vi "4461 - Create IO Channels Parallel.vi"(6 "AI Buffer Size (s)":i32=10, 8 "sampling info":cluster{"Fs":dbl, "#s":dbl}, 9 "AO":T1={"AO amp (V)"=[0.1, 0.09, 0.08, 0.07, 0.06, 0.05, 0.04, 0.03], "AO DC (V)"=[0.0, 0.0, 0.0, 0.0, 0.0, 0.0, 0.0, 0.0], "AO f (Hz)"=[13.0, 13.0, 13.0, 13.0, 13.0, 13.0, 13.0, 13.0], "AO phi (deg)"=[0.0, 0.0, 0.0, 0.0, 0.0, 0.0, 0.0, 0.0], "function"=[enum."Sine Wave", enum."Sine Wave", enum."Sine Wave", enum."Sine Wave", enum."Sine Wave", enum."Sine Wave", enum."Sine Wave", enum."Sine Wave"]} {"AO DC (V)" format="%#_6p"; "AO amp (V)" format="%#_6p"}, 10 "AO Configuration":T2(array[cluster])=[{"Output physical channels"="PXI1Slot2/ao0", "AO. Max"=0.1, "AO.Min"=-0.1}, {"Output physical channels"="", "AO. Max"=0.1, "AO.Min"=-0.1}], 11 "AI Configuration":T3(array[cluster])=[{"AI.Coupling"=10050, "AI.Max"=10.0, "AI.Min"=-10.0, "Input physical channels"="PXI1Slot2/ai0:1"}, {"AI.Coupling"=10050, "AI.Max"=10.0, "AI.Min"=-10.0, "Input physical channels"="PXI1Slot3/ai0:3"}, {"AI.Coupling"=10050, "AI.Max"=10.0, "AI.Min"=-10.0, "Input physical channels"=""}] {"AI.Coupling" items=["AC"=10045, "DC"=10050, "GND"=10066]}) -> (2 "AO Task":refnum<k21>[](array[refnum]), 3 "AI task":refnum<k21>[](array[refnum]), 4 "phase log":dbl[](array[numeric])=[0.99999999999938, 0.99999999999938], 5 "appended array":errorcluster[][](array[cluster]))   [LabVIEW 2013]
uses:
  <vilib>/DAQmx/configure/timing.llb/DAQmx Timing (Sample Clock).vi
  <vilib>/DAQmx/create/channels.llb/DAQmx Create Channel (AI-Voltage-Basic).vi
  <vilib>/DAQmx/write.llb/DAQmx Write (Analog 1D Wfm NChan NSamp).vi
  <resource>/objmgr/daqmx.rc
  <vilib>/DAQmx/configure/trigger.llb/DAQmx Start Trigger (Digital Edge).vi
  <vilib>/DAQmx/create/channels.llb/DAQmx Create Channel (AO-Voltage-Basic).vi
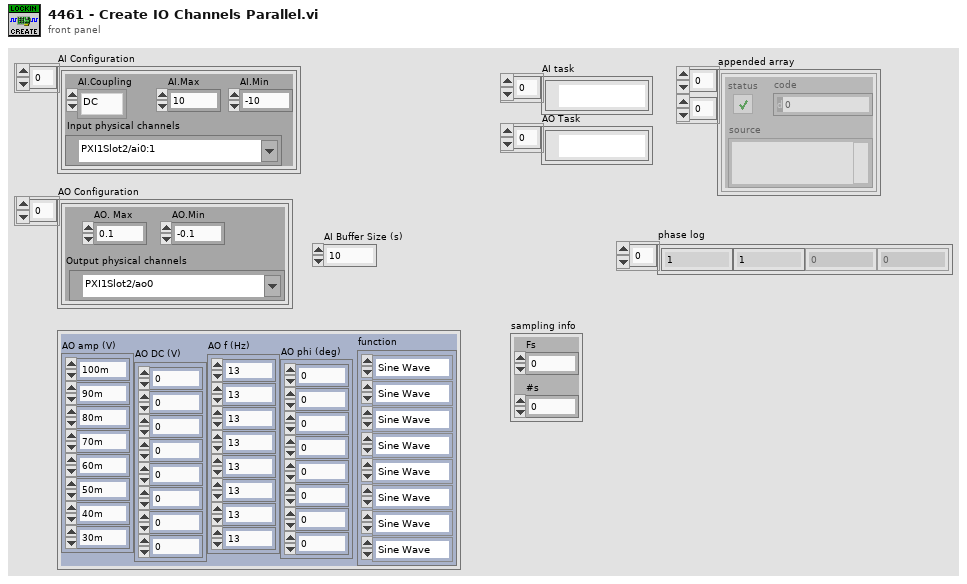
[diagram p1: front panel]
types:
  T1 = cluster{"AO amp (V)":dbl[], "AO DC (V)":dbl[], "AO f (Hz)":dbl[], "AO phi (deg)":dbl[], "function":enum16{"Sine Wave", "Triangle Wave", "Square Wave", "Sawtooth Wave"}[]}
  T2 = cluster{"Output physical channels":tag, "AO. Max":dbl, "AO.Min":dbl}[]
  T3 = cluster{"AI.Coupling":i32, "AI.Max":dbl, "AI.Min":dbl, "Input physical channels":tag}[]
  T4 = cluster{"AI.Coupling":i32, "AI.Max":dbl, "AI.Min":dbl, "Input physical channels":tag}
  T5 = cluster{"Output physical channels":tag, "AO. Max":dbl, "AO.Min":dbl}
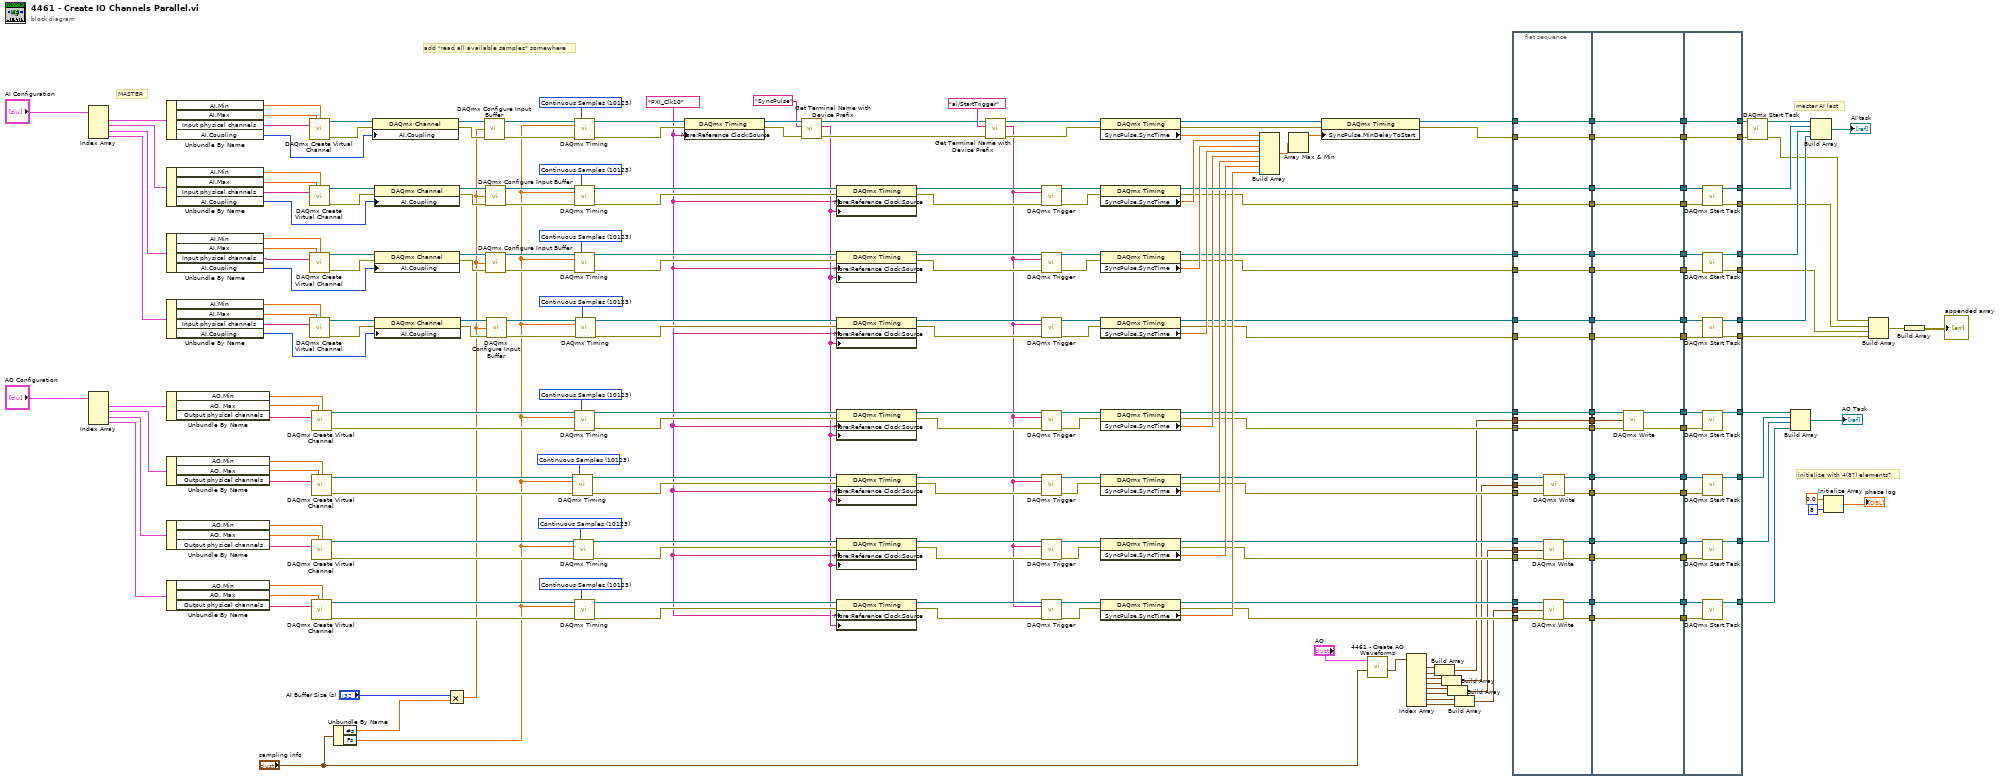
[diagram p0: block diagram]
diagram:
  w23 = tag "PXI_Clk10" ("RefClk.Src")
  w96 = 10123 items=["Finite Samples"=10178, "Continuous Samples"=10123] ("sample mode")
  w111 = 10123 items=["Finite Samples"=10178, "Continuous Samples"=10123] ("sample mode")
  w120 = 10123 items=["Finite Samples"=10178, "Continuous Samples"=10123] ("sample mode")
  w134 = 10123 items=["Finite Samples"=10178, "Continuous Samples"=10123] ("sample mode")
  w161 = 10123 items=["Finite Samples"=10178, "Continuous Samples"=10123] ("sample mode")
  w177 = 10123 items=["Finite Samples"=10178, "Continuous Samples"=10123] ("sample mode")
  w190 = 10123 items=["Finite Samples"=10178, "Continuous Samples"=10123] ("sample mode")
  w229 = 10123 items=["Finite Samples"=10178, "Continuous Samples"=10123] ("sample mode")
  # "master AI last"
  # "initialize with 4(8?) elements?"
  # "add \"read all available samples\" somewhere"
  # "MASTER"
  n1 = Index Array(array="AI Configuration") -> (element #1=w230:T4, element #2=w191:T4, element #3=w154:T4, element #4=w153:T4)  [unwired: 4 in]
  n2 = Index Array(array="AO Configuration") -> (element #1=w138:T5, element #2=w89:T5, element #3=w90:T5, element #4=w91:T5)  [unwired: 4 in]
  n3 = Unbundle By Name(w230) -> ("AI.Min"=w202:dbl, "AI.Max"=w203:dbl, "Input physical channels"=w214:tag, "AI.Coupling"=w201:i32)
  n4 = Unbundle By Name(w191) -> ("AI.Min"=w198:dbl, "AI.Max"=w197:dbl, "Input physical channels"=w192:tag, "AI.Coupling"=w199:i32)
  n5 = Unbundle By Name(w154) -> ("AI.Min"=w170:dbl, "AI.Max"=w171:dbl, "Input physical channels"=w176:tag, "AI.Coupling"=w169:i32)
  n6 = Unbundle By Name(w153) -> ("AI.Min"=w167:dbl, "AI.Max"=w166:dbl, "Input physical channels"=w162:tag, "AI.Coupling"=w168:i32)
  n7 = Unbundle By Name(w138) -> ("AO.Min"=w135:dbl, "AO. Max"=w136:dbl, "Output physical channels"=w137:tag)
  n8 = Unbundle By Name(w89) -> ("AO.Min"=w118:dbl, "AO. Max"=w117:dbl, "Output physical channels"=w116:tag)
  n9 = Unbundle By Name(w90) -> ("AO.Min"=w113:dbl, "AO. Max"=w114:dbl, "Output physical channels"=w115:tag)
  n10 = Unbundle By Name(w91) -> ("AO.Min"=w94:dbl, "AO. Max"=w93:dbl, "Output physical channels"=w92:tag)
  n11 = call-poly <vilib>:"DAQmx Create Virtual Channel.vi"("maximum value"=w203, "minimum value"=w202, "physical channels"=w214) -> ("task out"=w213:refnum<k21>, "error out"=w212:errorcluster)  [unwired: 11 in]
  n12 = call-poly <vilib>:"DAQmx Create Virtual Channel.vi"("maximum value"=w197, "minimum value"=w198, "physical channels"=w192) -> ("task out"=w193:refnum<k21>, "error out"=w194:errorcluster)  [unwired: 11 in]
  n13 = call-poly <vilib>:"DAQmx Create Virtual Channel.vi"("maximum value"=w171, "minimum value"=w170, "physical channels"=w176) -> ("task out"=w175:refnum<k21>, "error out"=w174:errorcluster)  [unwired: 11 in]
  n14 = call-poly <vilib>:"DAQmx Create Virtual Channel.vi"("maximum value"=w166, "minimum value"=w167, "physical channels"=w162) -> ("task out"=w163:refnum<k21>, "error out"=w164:errorcluster)  [unwired: 11 in]
  n15 = call-poly <vilib>:"DAQmx Create Virtual Channel.vi"("maximum value"=w136, "minimum value"=w135, "physical channels"=w137) -> ("task out"=w21:refnum<k21>, "error out"=w20:errorcluster)  [unwired: 11 in]
  n16 = call-poly <vilib>:"DAQmx Create Virtual Channel.vi"("maximum value"=w117, "minimum value"=w118, "physical channels"=w116) -> ("task out"=w119:refnum<k21>, "error out"=w121:errorcluster)  [unwired: 11 in]
  n17 = call-poly <vilib>:"DAQmx Create Virtual Channel.vi"("maximum value"=w114, "minimum value"=w113, "physical channels"=w115) -> ("task out"=w112:refnum<k21>, "error out"=w110:errorcluster)  [unwired: 11 in]
  n18 = call-poly <vilib>:"DAQmx Create Virtual Channel.vi"("maximum value"=w93, "minimum value"=w94, "physical channels"=w92) -> ("task out"=w95:refnum<k21>, "error out"=w97:errorcluster)  [unwired: 11 in]
  n19 = Unbundle By Name("sampling info") -> ("#s"=w2:dbl, "Fs"=w1:dbl)
  n20 = property class="DAQmx Channel"(reference=w213, error in=w212, "AI.Coupling"=w201) -> (reference out=w211:refnum<k21>, error out=w210:errorcluster)
  n21 = property class="DAQmx Channel"(reference=w193, error in=w194, "AI.Coupling"=w199) -> (reference out=w195:refnum<k21>, error out=w196:errorcluster)
  n22 = property class="DAQmx Channel"(reference=w175, error in=w174, "AI.Coupling"=w169) -> (reference out=w173:refnum<k21>, error out=w172:errorcluster)
  n23 = property class="DAQmx Channel"(reference=w163, error in=w164, "AI.Coupling"=w168) -> (reference out=w165:refnum<k21>, error out=w28:errorcluster)
  n24 = Multiply(x="AI Buffer Size (s)", y=w2) -> (x*y=w7:dbl)
  n25 = call <vilib>:"DAQmx Configure Input Buffer.vi"("task/channels in"=w211, "buffer size (in samples per channel)"=w7, "error in"=w210) -> ("task out"=w209:refnum<k21>, "error out"=w208:errorcluster)  [unwired: 11 in]
  n26 = call <vilib>:"DAQmx Configure Input Buffer.vi"("task/channels in"=w195, "buffer size (in samples per channel)"=w7, "error in"=w196) -> ("task out"=w189:refnum<k21>, "error out"=w188:errorcluster)  [unwired: 11 in]
  n27 = call <vilib>:"DAQmx Configure Input Buffer.vi"("task/channels in"=w173, "buffer size (in samples per channel)"=w7, "error in"=w172) -> ("task out"=w178:refnum<k21>, "error out"=w179:errorcluster)  [unwired: 11 in]
  n28 = call <vilib>:"DAQmx Configure Input Buffer.vi"("task/channels in"=w165, "buffer size (in samples per channel)"=w7, "error in"=w28) -> ("task out"=w160:refnum<k21>, "error out"=w159:errorcluster)  [unwired: 11 in]
  n29 = call-poly <vilib>:"DAQmx Timing.vi"("task/channels in"=w119, "sample mode"=w120, "rate"=w1, "error in"=w121) -> ("task out"=w123:refnum<k21>, "error out"=w124:errorcluster)  [unwired: 10 in]
  n30 = call-poly <vilib>:"DAQmx Timing.vi"("task/channels in"=w112, "sample mode"=w111, "rate"=w1, "error in"=w110) -> ("task out"=w108:refnum<k21>, "error out"=w107:errorcluster)  [unwired: 10 in]
  n31 = call-poly <vilib>:"DAQmx Timing.vi"("task/channels in"=w209, "sample mode"=w229, "rate"=w1, "error in"=w208) -> ("task out"=w228:refnum<k21>, "error out"=w200:errorcluster)  [unwired: 10 in]
  n32 = call-poly <vilib>:"DAQmx Timing.vi"("task/channels in"=w189, "sample mode"=w190, "rate"=w1, "error in"=w188) -> ("task out"=w187:refnum<k21>, "error out"=w186:errorcluster)  [unwired: 10 in]
  n33 = call-poly <vilib>:"DAQmx Timing.vi"("task/channels in"=w178, "sample mode"=w177, "rate"=w1, "error in"=w179) -> ("task out"=w180:refnum<k21>, "error out"=w181:errorcluster)  [unwired: 10 in]
  n34 = call-poly <vilib>:"DAQmx Timing.vi"("task/channels in"=w21, "sample mode"=w134, "rate"=w1, "error in"=w20) -> ("task out"=w132:refnum<k21>, "error out"=w131:errorcluster)  [unwired: 10 in]
  n35 = call-poly <vilib>:"DAQmx Timing.vi"("task/channels in"=w95, "sample mode"=w96, "rate"=w1, "error in"=w97) -> ("task out"=w99:refnum<k21>, "error out"=w100:errorcluster)  [unwired: 10 in]
  n36 = call-poly <vilib>:"DAQmx Timing.vi"("task/channels in"=w160, "sample mode"=w161, "rate"=w1, "error in"=w159) -> ("task out"=w158:refnum<k21>, "error out"=w157:errorcluster)  [unwired: 10 in]
  n37 = property class="DAQmx Timing"(reference=w228, error in=w200, "More:Reference Clock:Source"=w23) -> (reference out=w27:refnum<k21>, error out=w26:errorcluster)
  n38 = call "Get Terminal Name with Device Prefix.vi"("error in (no error)"=w26, "Local Terminal Name"="SyncPulse", "task/channels in"=w27) -> ("error out"=w223:errorcluster, "Terminal Name with Device Prefix"=w24:tag, "task out"=w224:refnum<k21>)  [unwired: 6 in]
  n39 = property class="DAQmx Timing"(reference=w187, error in=w186, "More:Reference Clock:Source"=w23, "More:Synchronization Pulse:Source"=w24) -> (reference out=w185:refnum<k21>, error out=w184:errorcluster)
  n40 = property class="DAQmx Timing"(reference=w180, error in=w181, "More:Reference Clock:Source"=w23, "More:Synchronization Pulse:Source"=w24) -> (reference out=w182:refnum<k21>, error out=w183:errorcluster)
  n41 = property class="DAQmx Timing"(reference=w158, error in=w157, "More:Reference Clock:Source"=w23, "More:Synchronization Pulse:Source"=w24) -> (reference out=w156:refnum<k21>, error out=w155:errorcluster)
  n42 = property class="DAQmx Timing"(reference=w132, error in=w131, "More:Reference Clock:Source"=w23, "More:Synchronization Pulse:Source"=w24) -> (reference out=w133:refnum<k21>, error out=w130:errorcluster)
  n43 = property class="DAQmx Timing"(reference=w123, error in=w124, "More:Reference Clock:Source"=w23, "More:Synchronization Pulse:Source"=w24) -> (reference out=w122:refnum<k21>, error out=w125:errorcluster)
  n44 = property class="DAQmx Timing"(reference=w108, error in=w107, "More:Reference Clock:Source"=w23, "More:Synchronization Pulse:Source"=w24) -> (reference out=w109:refnum<k21>, error out=w106:errorcluster)
  n45 = property class="DAQmx Timing"(reference=w99, error in=w100, "More:Reference Clock:Source"=w23, "More:Synchronization Pulse:Source"=w24) -> (reference out=w98:refnum<k21>, error out=w101:errorcluster)
  n46 = call "Get Terminal Name with Device Prefix.vi"("error in (no error)"=w223, "Local Terminal Name"="ai/StartTrigger", "task/channels in"=w224) -> ("error out"=w221:errorcluster, "Terminal Name with Device Prefix"=w84:tag, "task out"=w222:refnum<k21>)  [unwired: 6 in]
  n47 = call-poly <vilib>:"DAQmx Trigger.vi"("task/channels in"=w185, "source"=w84, "error in"=w184) -> ("task out"=w150:refnum<k21>, "error out"=w149:errorcluster)  [unwired: 11 in]
  n48 = call-poly <vilib>:"DAQmx Trigger.vi"("task/channels in"=w182, "source"=w84, "error in"=w183) -> ("task out"=w151:refnum<k21>, "error out"=w148:errorcluster)  [unwired: 11 in]
  n49 = call-poly <vilib>:"DAQmx Trigger.vi"("task/channels in"=w156, "source"=w84, "error in"=w155) -> ("task out"=w152:refnum<k21>, "error out"=w147:errorcluster)  [unwired: 11 in]
  n50 = call-poly <vilib>:"DAQmx Trigger.vi"("task/channels in"=w133, "source"=w84, "error in"=w130) -> ("task out"=w129:refnum<k21>, "error out"=w128:errorcluster)  [unwired: 11 in]
  n51 = call-poly <vilib>:"DAQmx Trigger.vi"("task/channels in"=w122, "source"=w84, "error in"=w125) -> ("task out"=w126:refnum<k21>, "error out"=w127:errorcluster)  [unwired: 11 in]
  n52 = call-poly <vilib>:"DAQmx Trigger.vi"("task/channels in"=w109, "source"=w84, "error in"=w106) -> ("task out"=w105:refnum<k21>, "error out"=w104:errorcluster)  [unwired: 11 in]
  n53 = call-poly <vilib>:"DAQmx Trigger.vi"("task/channels in"=w98, "source"=w84, "error in"=w101) -> ("task out"=w102:refnum<k21>, "error out"=w103:errorcluster)  [unwired: 11 in]
  n54 = property class="DAQmx Timing"(reference=w222, error in=w221) -> (reference out=w218:refnum<k21>, error out=w219:errorcluster, "SyncPulse.SyncTime"=w220:dbl)
  n55 = property class="DAQmx Timing"(reference=w150, error in=w149) -> (reference out=w140:refnum<k21>, error out=w75:errorcluster, "SyncPulse.SyncTime"=w145:dbl)
  n56 = property class="DAQmx Timing"(reference=w151, error in=w148) -> (reference out=w81:refnum<k21>, error out=w72:errorcluster, "SyncPulse.SyncTime"=w144:dbl)
  n57 = property class="DAQmx Timing"(reference=w152, error in=w147) -> (reference out=w78:refnum<k21>, error out=w69:errorcluster, "SyncPulse.SyncTime"=w143:dbl)
  n58 = property class="DAQmx Timing"(reference=w129, error in=w128) -> (reference out=w66:refnum<k21>, error out=w57:errorcluster, "SyncPulse.SyncTime"=w88:dbl)
  n59 = property class="DAQmx Timing"(reference=w126, error in=w127) -> (reference out=w63:refnum<k21>, error out=w55:errorcluster, "SyncPulse.SyncTime"=w87:dbl)
  n60 = property class="DAQmx Timing"(reference=w105, error in=w104) -> (reference out=w60:refnum<k21>, error out=w52:errorcluster, "SyncPulse.SyncTime"=w86:dbl)
  n61 = property class="DAQmx Timing"(reference=w102, error in=w103) -> (reference out=w49:refnum<k21>, error out=w46:errorcluster, "SyncPulse.SyncTime"=w85:dbl)
  n62 = Build Array(w220, w145, w144, w143, w88, w87, w86, w85) -> (w217:dbl[])
  n63 = Array Max & Min(array=w217) -> (max value=w146:dbl)  [unwired: 3 out]
  n64 = property class="DAQmx Timing"(reference=w218, error in=w219, "SyncPulse.MinDelayToStart"=w146) -> (reference out=w215:refnum<k21>, error out=w216:errorcluster)
  n65 = call "4461 - Create AO Waveforms.vi"("sampling info"="sampling info", "AO"="AO") -> ("AO Array"=w5:waveform(dbl)[])  [unwired: 7 in, 2 out]
  n66 = Index Array(array=w5) -> (element #1=w8:waveform(dbl), element #2=w19:waveform(dbl), element #3=w18:waveform(dbl), element #4=w17:waveform(dbl), element #5=w16:waveform(dbl), element #6=w15:waveform(dbl), element #7=w14:waveform(dbl), element #8=w13:waveform(dbl))  [unwired: 8 in]
  n67 = Build Array(w8, w19) -> (w12:waveform(dbl)[])
  n68 = Build Array(w18, w17) -> (w11:waveform(dbl)[])
  n69 = Build Array(w16, w15) -> (w10:waveform(dbl)[])
  n70 = Build Array(w14, w13) -> (w9:waveform(dbl)[])
  n71 = flat-sequence {
    tunnel: w216 -> [w259]
    tunnel: w215 -> [w260]
    tunnel: [w260] -> w234
    tunnel: [w259] -> w233
    tunnel: [w258] -> w141
    tunnel: w140 -> [w258]
    tunnel: [w257] -> w82
    tunnel: w81 -> [w257]
    tunnel: [w256] -> w79
    tunnel: w78 -> [w256]
    tunnel: [w255] -> w76
    tunnel: w75 -> [w255]
    tunnel: [w254] -> w73
    tunnel: w72 -> [w254]
    tunnel: [w253] -> w70
    tunnel: w69 -> [w253]
    tunnel: [w252] -> w67
    tunnel: w66 -> [w252]
    tunnel: [w240] -> w64
    tunnel: w63 -> [w241]
    tunnel: [w244] -> w61
    tunnel: w60 -> [w243]
    tunnel: [w251] -> w58
    tunnel: w57 -> [w251]
    tunnel: w55 -> [w242]
    tunnel: [w245] -> w53
    tunnel: w52 -> [w246]
    tunnel: [w247] -> w50
    tunnel: w49 -> [w250]
    tunnel: [w248] -> w47
    tunnel: w46 -> [w249]
    tunnel: [w239] -> w45
    tunnel: [w238] -> w36
    tunnel: w12 -> [w238]
    tunnel: w11 -> [w237]
    tunnel: w10 -> [w236]
    tunnel: w9 -> [w235]
    tunnel: [w279] -> w232
    tunnel: [w278] -> w231
    tunnel: w234 -> [w279]
    tunnel: w233 -> [w278]
    tunnel: [w277] -> w142
    tunnel: w141 -> [w277]
    tunnel: [w276] -> w83
    tunnel: w82 -> [w276]
    tunnel: [w275] -> w80
    tunnel: w79 -> [w275]
    tunnel: [w274] -> w77
    tunnel: w76 -> [w274]
    tunnel: [w273] -> w74
    tunnel: w73 -> [w273]
    tunnel: [w272] -> w71
    tunnel: w70 -> [w272]
    tunnel: [w264] -> w68
    tunnel: w67 -> [w265]
    tunnel: [w271] -> w65
    tunnel: w64 -> [w271]
    tunnel: [w270] -> w62
    tunnel: w61 -> [w270]
    tunnel: [w263] -> w59
    tunnel: w58 -> [w262]
    tunnel: [w269] -> w56
    tunnel: [w268] -> w54
    tunnel: w53 -> [w268]
    tunnel: [w267] -> w51
    tunnel: w50 -> [w267]
    tunnel: [w266] -> w48
    tunnel: w47 -> [w266]
    tunnel: w45 -> [w269]
    tunnel: w36 -> [w261]
    tunnel: [w305] -> w227
    tunnel: [w304] -> w226
    tunnel: w232 -> [w305]
    tunnel: w231 -> [w304]
    tunnel: w142 -> [w303]
    tunnel: w83 -> [w302]
    tunnel: w80 -> [w301]
    tunnel: w77 -> [w300]
    tunnel: w74 -> [w299]
    tunnel: w71 -> [w298]
    tunnel: w68 -> [w297]
    tunnel: w65 -> [w296]
    tunnel: w62 -> [w295]
    tunnel: w59 -> [w294]
    tunnel: w56 -> [w293]
    tunnel: w54 -> [w292]
    tunnel: w51 -> [w291]
    tunnel: w48 -> [w290]
    tunnel: [w289] -> w44
    tunnel: [w288] -> w43
    tunnel: [w287] -> w42
    tunnel: [w286] -> w41
    tunnel: [w285] -> w40
    tunnel: [w284] -> w39
    tunnel: [w283] -> w38
    tunnel: [w282] -> w35
    tunnel: [w281] -> w32
    tunnel: [w280] -> w34
    frame #0 {
      n72 = call-poly <vilib>:"DAQmx Write.vi"("task/channels in"=w243, "data"=w236, "error in"=w246) -> ("task out"=w244:refnum<k21>, "error out"=w245:errorcluster)  [unwired: 10 in, 1 out]
      n73 = call-poly <vilib>:"DAQmx Write.vi"("task/channels in"=w250, "data"=w235, "error in"=w249) -> ("task out"=w247:refnum<k21>, "error out"=w248:errorcluster)  [unwired: 10 in, 1 out]
      n74 = call-poly <vilib>:"DAQmx Write.vi"("task/channels in"=w241, "data"=w237, "error in"=w242) -> ("task out"=w240:refnum<k21>, "error out"=w239:errorcluster)  [unwired: 10 in, 1 out]
    }
    frame #1 {
      n75 = call-poly <vilib>:"DAQmx Write.vi"("task/channels in"=w265, "data"=w261, "error in"=w262) -> ("task out"=w264:refnum<k21>, "error out"=w263:errorcluster)  [unwired: 10 in, 1 out]
    }
    frame #2 {
      n76 = call <vilib>:"DAQmx Start Task.vi"("task/channels in"=w303, "error in"=w300) -> ("task out"=w289:refnum<k21>, "error out"=w282:errorcluster)  [unwired: 12 in]
      n77 = call <vilib>:"DAQmx Start Task.vi"("task/channels in"=w302, "error in"=w299) -> ("task out"=w288:refnum<k21>, "error out"=w281:errorcluster)  [unwired: 12 in]
      n78 = call <vilib>:"DAQmx Start Task.vi"("task/channels in"=w301, "error in"=w298) -> ("task out"=w287:refnum<k21>, "error out"=w280:errorcluster)  [unwired: 12 in]
      n79 = call <vilib>:"DAQmx Start Task.vi"("task/channels in"=w297, "error in"=w294) -> ("task out"=w286:refnum<k21>)  [unwired: 12 in, 1 out]
      n80 = call <vilib>:"DAQmx Start Task.vi"("task/channels in"=w296, "error in"=w293) -> ("task out"=w285:refnum<k21>)  [unwired: 12 in, 1 out]
      n81 = call <vilib>:"DAQmx Start Task.vi"("task/channels in"=w295, "error in"=w292) -> ("task out"=w284:refnum<k21>)  [unwired: 12 in, 1 out]
      n82 = call <vilib>:"DAQmx Start Task.vi"("task/channels in"=w291, "error in"=w290) -> ("task out"=w283:refnum<k21>)  [unwired: 12 in, 1 out]
    }
  }
  n83 = call <vilib>:"DAQmx Start Task.vi"("task/channels in"=w227, "error in"=w226) -> ("task out"=w206:refnum<k21>, "error out"=w22:errorcluster)  [unwired: 12 in]
  n84 = Build Array(w41, w40, w39, w38) -> (→"AO Task":refnum<k21>[])
  n85 = Build Array(w206, w44, w43, w42) -> (→"AI task":refnum<k21>[])
  n86 = Initialize Array(0.0 ("element"), 8 ("dimension size")) -> (→"phase log":dbl[])
  n87 = Build Array(w22, w35, w32, w34) -> (w33:errorcluster[])
  n88 = Build Array(w33) -> (→"appended array":errorcluster[][])
